vi "Error.vi"(8 "error in (no error)":errorcluster, 11 "Error Data":errorcluster) -> (0 "error out":errorcluster)   [LabVIEW 2017, in "Error.lvlib"]
doc: "Go to error state"
uses:
  Error.lvlib
  ctl/MainData.ctl
  ctl/MainStates.ctl
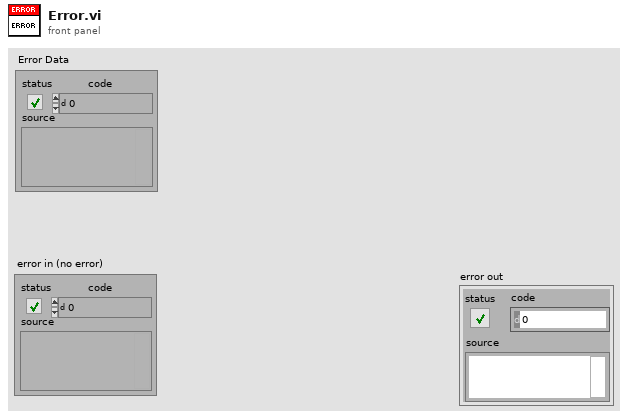
[diagram p1: front panel]
types:
  T1 = typedef "Error.lvlib/MainStates.ctl" = enum16{"Timeout", "Error", "Exit", "Init"}
  T2 = typedef "Error.lvlib/MainData.ctl" = cluster{"State":T1, "Variant":variant}
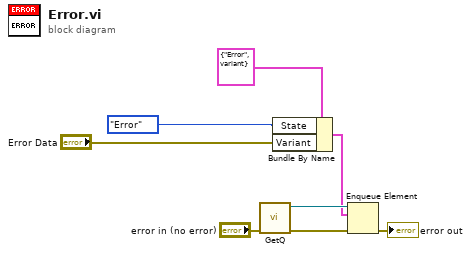
[diagram p0: block diagram]
diagram:
  n1 = call "GetQ.vi"("error in (no error)"="error in (no error)") -> ("error out"=w7:errorcluster, "Q out"=w8:refnum<queue>)  [unwired: 9 in]
  n2 = Bundle By Name(cluster=T2 {"State"=enum."Error", "Variant"=variant} ("Data"), "State"=MainStates."Error", "Variant"="Error Data") -> (w4:T2)
  n3 = Enqueue Element(queue=w8, element=w4, error in (no error)=w7) -> (error out=→"error out":errorcluster)  [unwired: 1 in, 2 out]
